vi "terminar.vi"(1 "Cliente in":refnum<class "Cliente.lvclass">) -> (0 "Cliente out":refnum<class "Cliente.lvclass">)   [LabVIEW 2015, in "Cliente.lvclass"]
uses:
  Cliente.lvclass
  Cliente.lvclass/Cliente.ctl
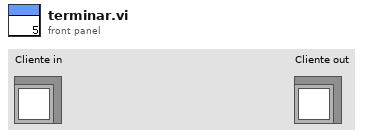
[diagram p1: front panel]
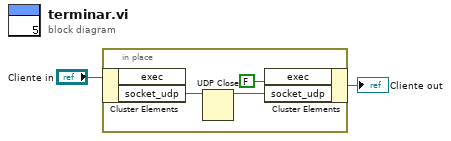
[diagram p0: block diagram]
diagram:
  n1 = in-place {
    n2 = in-place-cluster #1("Cliente in") -> ("socket_udp"=w4:refnum<k16>)  [unwired: 1 out]
    n3 = UDP Close(connection ID=w4) -> (connection ID out=w3:refnum<k16>)  [unwired: 1 in, 1 out]
    n4 = in-place-cluster #1("exec"=FALSE, "socket_udp"=w3) -> (→"Cliente out":refnum<class "Cliente.lvclass">)
  }
